vi "Modify_VIPB_LabVIEW_Version.vi"   [LabVIEW 2021]
uses:
  <vilib>/Wiresmith Technology/G CLI/CLI Class/CLI.lvclass
types:
  T1 = enum16{"open", "replace", "create", "open or create", "replace or create", "replace or create with confirmation"}
  T2 = enum32{"Invalid", "Standard", "Closed", "Hidden", "Minimized", "Maximized"}
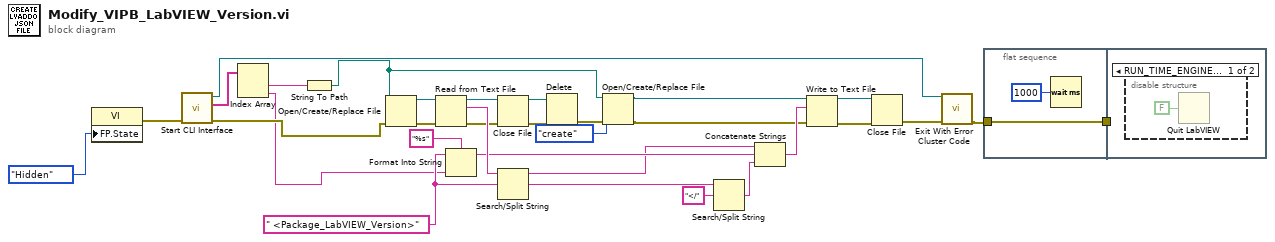
[diagram p0: block diagram]
diagram:
  w23 = " <Package_LabVIEW_Version>" ("search string")
  n1 = property class="VI"("FP.State"=T2."Hidden" ("Front Panel Window:State")) -> (error out=w30:errorcluster)  [unwired: 2 in, 1 out]
  n2 = call <vilib>:"Start CLI Interface.vi"("error in (no error)"=w30) -> ("error out"=w2:errorcluster, "Custom Parameters"=w15:string[], "CLI out"=w12:refnum<class "CLI.lvclass">)  [unwired: 7 in, 1 out]
  n3 = Index Array(array=w15) -> (element #1=w14:string, element #2=w1:string)  [unwired: 2 in]
  n4 = String To Path(string=w14) -> (path=w3:path)
  n5 = Open/Create/Replace File(file path (use dialog)=w3, error in=w2) -> (refnum out=w27:refnum<file>, error out=w28:errorcluster)  [unwired: 4 in, 1 out]
  n6 = Read from Text File(file (use dialog)=w27, error in=w28) -> (refnum out=w11:refnum<file>, text=w26:string, error out=w10:errorcluster)  [unwired: 2 in, 1 out]
  n7 = Format Into String(format string="%s", initial string=w23, w1) -> (resulting string=w21:string)  [unwired: 1 in, 1 out]
  n8 = Close File(refnum=w11, error in=w10) -> (path=w8:path, error out=w9:errorcluster)
  n9 = Search/Split String(string=w26, search string/char (-)=w23) -> (substring before match=w19:string, match + rest of string=w25:string)  [unwired: 1 in, 1 out]
  n10 = Delete(path (use dialog)=w8, error in=w9) -> (error out=w7:errorcluster)  [unwired: 3 in, 2 out]
  n11 = Open/Create/Replace File(file path (use dialog)=w3, error in=w7, operation (0:open)=T1."create") -> (refnum out=w6:refnum<file>, error out=w5:errorcluster)  [unwired: 3 in, 1 out]
  n12 = Search/Split String(string=w25, search string/char (-)="</") -> (match + rest of string=w20:string)  [unwired: 1 in, 2 out]
  n13 = Concatenate Strings(w19, w21, w20) -> (w18:string)
  n14 = Write to Text File(file (use dialog)=w6, text=w18, error in=w5) -> (refnum out=w16:refnum<file>, error out=w17:errorcluster)  [unwired: 1 in, 1 out]
  n15 = Close File(refnum=w16, error in=w17) -> (error out=w13:errorcluster)  [unwired: 1 out]
  n16 = call <vilib>:"Exit With Error Cluster Code.vi"("error in (no error)"=w13, "CLI in"=w12) -> ("error out"=w29:errorcluster)  [unwired: 9 in]
  n17 = flat-sequence {
    tunnel: w29 -> [w34]
    tunnel: [w34] -> w32
    tunnel: w32 -> [_]
    frame #0 {
      n18 = Wait (ms)(milliseconds to wait=u32 1000) -> ()  [unwired: 1 out]
    }
    frame #1 {
      n19 = disable-structure shown="RUN_TIME_ENGINE==True" {
        frame condition #0 {
          n20 = Quit LabVIEW(quit? (T)=FALSE) -> ()
        }
        frame condition #1 (active) {
        }
      }
    }
  }
